vi "subVI verify state_demoinfocom.vi"(10 "Enum":enum16{"State 1"}(ring), 11 "Channel in":T1) -> (2 "State 1 Indicator":bool, 3 "element":enum16{"State 1", "State 2", "State 3"}(ring))   [LabVIEW 2021]
uses:
  <extravilib>/ChannelInstances/Tag-u16[State 1,State 2,State 3]/))Channel.ctl
  <extravilib>/ChannelInstances/Tag-u16[State 1,State 2,State 3]/Read With Abort.vi
  <extravilib>/ChannelInstances/Tag-u16[State 1,State 2,State 3]/EndpointRead.vi
  <extravilib>/ChannelInstances/Tag-u16[State 1,State 2,State 3].lvlib
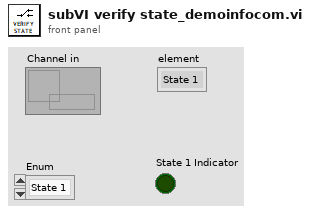
[diagram p1: front panel]
types:
  T1 = typedef "Tag-u16[State 1,State 2,State 3].lvlib/))Channel.ctl" = refnum<queue>
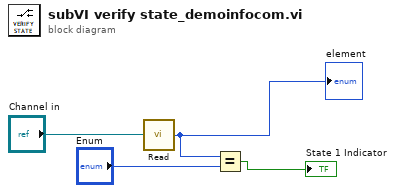
[diagram p0: block diagram]
diagram:
  n1 = call <extravilib>:"Read.vi"("channel"="Channel in") -> ("element"=w2:enum16{"State 1", "State 2", "State 3"})  [unwired: 1 in, 1 out]
  "element" <- w2
  n2 = Equal?(x=w2, y="Enum") -> (x = y?=→"State 1 Indicator":bool)
